vi "TestAO.vi"() -> ()   [LabVIEW 2012]
uses:
  <vilib>/DAQmx/write.llb/DAQmx Write (Analog DBL 1Chan 1Samp).vi
  <vilib>/DAQmx/create/channels.llb/DAQmx Create Channel (AO-Voltage-Basic).vi
  <vilib>/DAQmx/miscellaneous.llb/DAQmx Fill In Error Info.vi
panel:
  in  "stop":bool
  in  "data":dbl format="%0.2f"
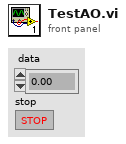
[diagram p1: front panel]
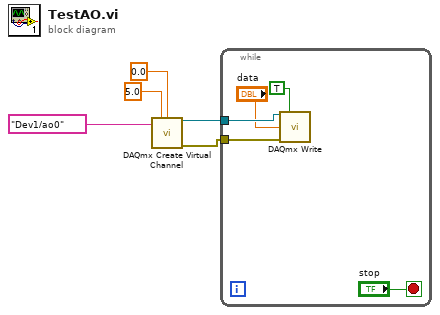
[diagram p0: block diagram]
diagram:
  n1 = call-poly <vilib>:"DAQmx Create Virtual Channel.vi"("maximum value"=5.0, "minimum value"=0.0, "physical channels"=tag "Dev1/ao0") -> ("task out"=w4:refnum<k21>, "error out"=w3:errorcluster)  [unwired: 11 in]
  n2 = while {
    tunnel: w4 -> [w10]
    tunnel: w3 -> [w8]
    stop <- "stop" stop-if-true
    n3 = call-poly <vilib>:"DAQmx Write.vi"("task/channels in"=w10, "auto start"=TRUE, "data"="data", "error in"=w8) -> ()  [unwired: 9 in, 3 out]
  }
